vi "Save Profile.vi"(8 "Key Binds":u16[](array[ring]) items=["No Function", "Gear Shift", "Direction Toggle", "Cube Up", "Cube Down", "LRamp Deploy", "RRamp Deploy", "LRamp Raise", "RRamp Raise"], 9 "Profile Name":string, 10 "Driver Pref":dbl[](array[numeric]), 11 "Output":bool) -> (0 "error out":errorcluster)   [LabVIEW 2018]
uses:
  <vilib>/Utility/file.llb/Write Delimited Spreadsheet (DBL).vi
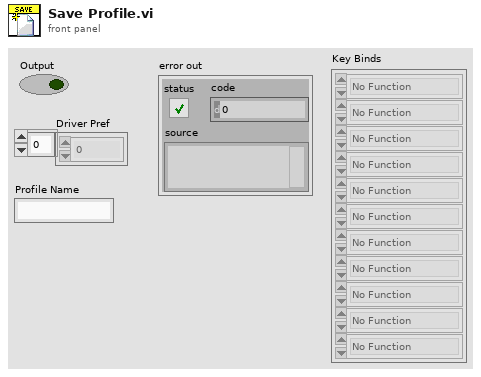
[diagram p1: front panel]
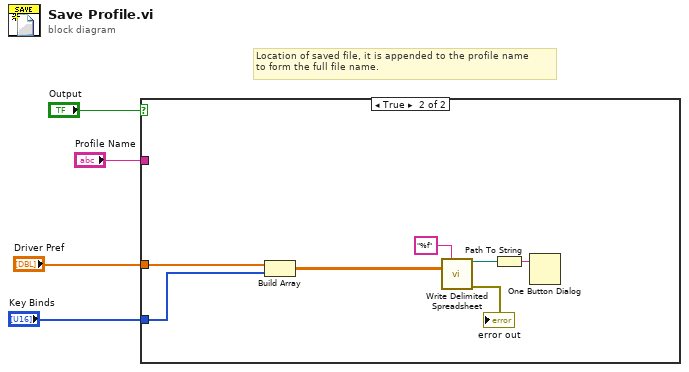
[diagram p0: block diagram]
diagram:
  # "Location of saved file, it is appended to the profile name \nto form the full file name."
  n1 = case shown="True" "Output" {
    tunnel: "Driver Pref" -> [_ w8]
    tunnel: "Profile Name" -> [_ _]
    tunnel: "Key Binds" -> [_ w7]
    frame False {
    }
    frame True {
      n2 = Build Array(w8, w7) -> (w6:dbl[][])
      n3 = call-poly <vilib>:"Write Delimited Spreadsheet.vi"("format (%.3f)"="%f", "2D data"=w6) -> ("new file path (Not A Path if cancelled)"=w5:path, "error out"=→"error out":errorcluster)  [unwired: 12 in]
      n4 = Path To String(path=w5) -> (string=w10:string)
      n5 = One Button Dialog(message=w10) -> ()  [unwired: 1 in, 1 out]
    }
  }
